vi "Run.vi"(8 "Error In":errorcluster, 10 "Abstract Syntax Tree":refnum<class "Root.lvclass">, 11 "Renderer In":refnum<class "Renderer.lvclass">) -> (0 "Error Out":errorcluster, 3 "Renderer Out":refnum<class "Renderer.lvclass">)   [LabVIEW 2018, in "Toolkit.lvlib" / "Renderer.lvclass"]
uses:
  Renderer.lvclass
  Nodes/Root/Root.lvclass
  Renderer.lvclass/Renderer.ctl
  Writers/Writer/Writer.lvclass
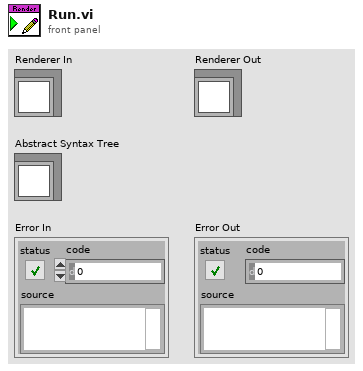
[diagram p1: front panel]
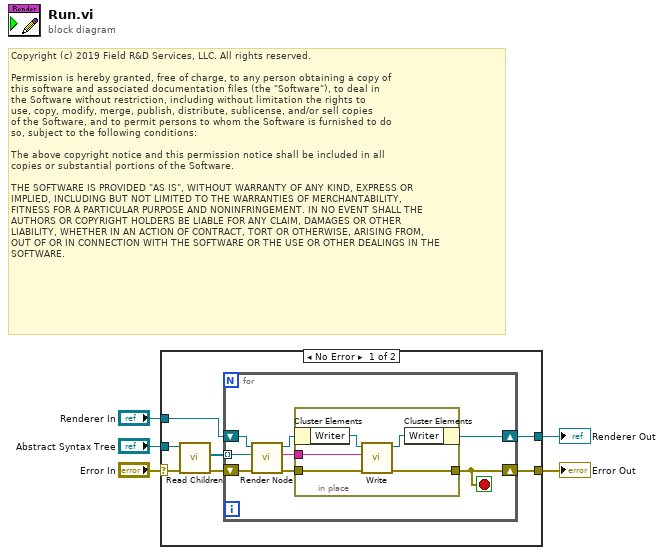
[diagram p0: block diagram]
diagram:
  # "Copyright (c) 2019 Field R&D Services, LLC. All rights reserved.\n\nPermission is hereby granted, free of charge, to any person obtaining a copy of\nthis software and associated documentation files (the \"Software\"), to deal in\nthe Software without restriction, including without limitation the rights to\nuse, copy, modify, merge, publish, distribute, sublicense, and/or sell copies\nof the Software, and to permit persons to whom the Software is furnished to do\nso, subject to the following conditions:\n\nThe above copyright notice and this permission notice shall be included in all\ncopies or substantial portions of the Software.\n\nTHE SOFTWARE IS PROVIDED \"AS IS\", WITHOUT WARRANTY OF ANY KIND, EXPRESS OR\nIMPLIED, INCLUDING BUT NOT LIMITED TO THE WARRANTIES OF MERCHANTABILITY,\nFITNESS FOR A PARTICULAR PURPOSE AND NONINFRINGEMENT. IN NO EVENT SHALL THE\nAUTHORS OR COPYRIGHT HOLDERS BE LIABLE FOR ANY CLAIM, DAMAGES OR OTHER\nLIABILITY, WHETHER IN AN ACTION OF CONTRACT, TORT OR OTHERWISE, ARISING FROM,\nOUT OF OR IN CONNECTION WITH THE SOFTWARE OR THE USE OR OTHER DEALINGS IN THE\nSOFTWARE."
  n1 = case shown="No Error" "Error In" {
    selector: "Error In" -> [w8 w27]
    tunnel: [w6 w27] -> w4
    tunnel: "Abstract Syntax Tree" -> [w9 _]
    tunnel: "Renderer In" -> [w10 w26]
    tunnel: [w7 w26] -> w1
    frame No Error {
      n2 = call-dynamic "Read Children.vi"("Error In"=w8, "Non-Terminal In"=w9) -> ("Error Out"=w11:errorcluster, "Children"=w12:refnum<class "Node.lvclass">[])  [unwired: 7 in, 1 out]
      n3 = for {
        tunnel: w12 -> [w18] mode=indexing
        shift-right: [w15] -> w6
        shift-left: w11 -> [w20]
        shift-right: [w13] -> w7
        shift-left: w10 -> [w16]
        stop <- w15 stop-if-true
        n4 = call-dynamic "Render Node.vi"("Error In"=w20, "Node"=w18, "Renderer In"=w16) -> ("Error Out"=w19:errorcluster, "Output"=w17:string, "Renderer Out"=w14:refnum<class "Renderer.lvclass">)  [unwired: 6 in]
        n5 = in-place {
          in-place-border: w19 -> [w25]
          in-place-border: w17 -> [w24]
          in-place-border: [w23] -> w15
          n6 = in-place-cluster #1(w14) -> ("Writer"=w22:refnum<class "Writer.lvclass">)
          n7 = call-dynamic "Write.vi"("Error In"=w25, "Content"=w24, "Writer In"=w22) -> ("Error Out"=w23:errorcluster, "Writer Out"=w21:refnum<class "Writer.lvclass">)  [unwired: 7 in]
          n8 = in-place-cluster #1("Writer"=w21) -> (w13:refnum<class "Renderer.lvclass">)
        }
      }
    }
    frame Error {
    }
  }
  "Error Out" <- w4
  "Renderer Out" <- w1
